vi "Select_Time.vi"(8 "error in (no error)":errorcluster, 9 "State In":T1=enum."Staged", 10 "Time Remaining in":dbl, 11 "Initial Recipe Time":dbl) -> (0 "error out":errorcluster, 3 "Time Remaining out":dbl)   [LabVIEW 2026]
uses:
  controls/System_Status.ctl
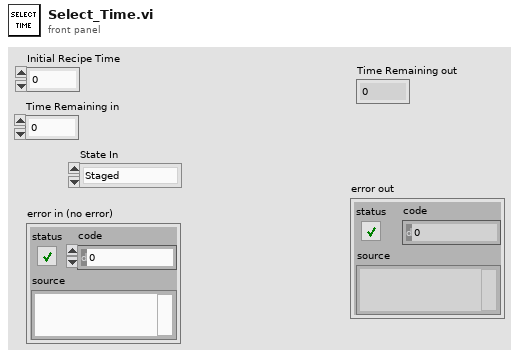
[diagram p1: front panel]
types:
  T1 = typedef "System_Status.ctl" = enum16{"Idle", "Staged", "Cooking", "Paused", "Buzzer Alert"}
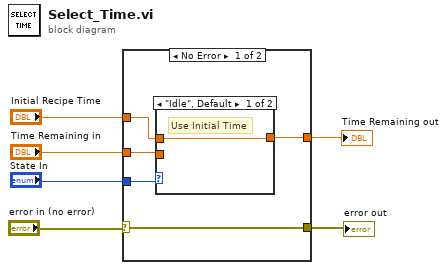
[diagram p0: block diagram]
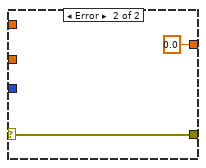
[diagram p3: hidden frame]
diagram:
  n1 = case shown="No Error" "error in (no error)" {
    selector: "error in (no error)" -> [w7 w15]
    tunnel: "Initial Recipe Time" -> [w11 _]
    tunnel: "Time Remaining in" -> [w10 _]
    tunnel: [w9 0.0 ("Time Remaining in")] -> w4
    tunnel: "State In" -> [w8 _]
    tunnel: [w7 w15] -> w1
    frame No Error {
      n2 = case shown="\"Idle\", Default" w8 {
        tunnel: w10 -> [_ w13]
        tunnel: [w12 w13] -> w9
        tunnel: w11 -> [w12 _]
        frame "Idle", Default {
          # "Use Initial Time"
        }
        frame "Staged" {
          # "Use Running Time"
        }
      }
    }
    frame Error {
    }
  }
  "Time Remaining out" <- w4
  "error out" <- w1
